vi "Lab7-PSK_Simulation_4PSK_Simple.vi"() -> ()   [LabVIEW 2013]
uses:
  <vilib>/picture/picture.llb/Draw True-Color Pixmap.vi
  <vilib>/addons/Modulation/Digital/General/MT Generate Bits (Galois, PN Order).vi
  <vilib>/addons/Modulation/Digital/General/MT Generate PSK System Parameters(M).vi
  <vilib>/addons/Modulation/Digital/General/MT Generate PSK Synchronization Parameters (bit array).vi
  <vilib>/addons/Modulation/Digital/General/MT Format Eye Diagram (complex).vi
  <vilib>/addons/Modulation/niDMT.lvlib
panel:
  in  "?":enum32{"Constellation Plot", "Eye Diagram"}(tab)
  out "Constellation Plot":T1(graph)=[{"constellation"=[-0.6843393450045908, -0.7188173867833647, -0.6862679721424542, -0.7297030487459608, -0.7159912856499204, 0.7221248350001428, -0.69319374455267, -0.7177933374862676, 0.6893145049073991, 0.7164949508669772, -0.7136233597527977, 0.7088022813066004, 0.7026806753460019, 0.6993908820448104, 0.7033303803758204, 0.7023239283689477, -0.7092821972958672, 0.7043694263023035, -0.71123073342578, -0.7063013580615412, 0.7025174893431778, -0.7079249457114573, 0.7056952690720733, -0.711060440916994, -0.7135916049305011, -0.7042966683375681, -0.7053639500078486, -0.7170793110386893, 0.7007122470722706, -0.7041907238690962, 0.7069307076270948, -0.7303032352912369, 0.7036742608538313, -0.7213763894899665, 0.6974920430188264, -0.6906276182534745, 0.7110338385529501, 0.707668395707459, 0.7066450908567875, 0.7156573983712801, 0.7058430026446071, 0.7226424194495579, -0.6941394170921843, 0.7153952742388731, -0.7061754291757949, 0.6989077999376425, 0.7322949703863137, -0.7277124364880128, 0.7152053555332901, -0.7144386806873485, 0.7122523333502172, -0.6946532350705298, -0.6977995339788963], "oversampled data"=[-0.6885507056398621, -0.6904021301332153, -0.701720009748651, 0.7230147663617461, 0.6792985003415442, 0.714980330495899, 0.7083798924531897, -0.7030264642885489, 0.7016069656212314, -0.6995735246622811, -0.7187083014951974, 0.718556461974981, -0.7154964369422703, -0.7143626925937305, -0.7168215682367294, 0.6901290658424636, 0.7193430662186729, 0.7021618219264352, -0.7044915371643418, 0.7010427354068245, 0.72862911894502, -0.6931780204687834, -0.7208414620302925, 0.6898461638663613, 0.7171050214665211, 0.7071101521691305, -0.7158811583840712, 0.7100771986297291, 0.7055043383295747, 0.7197934468495215, -0.7126751015343431, 0.699715799910657, 0.7071055136917425, 0.7000396806158872, 0.6959369636505729, 0.7171363071737368, 0.7097950846368283, 0.707670861017943, 0.6989567675175453, -0.7157042609479739, 0.7040676123623458, 0.7131191099779645, 0.7010491472655718, 0.7001052143691281, -0.7044803945850813, 0.6953086657664377, 0.7183481414573912, 0.7015721146800344, -0.6848840235343148, -0.712341720231345, 0.7005395668208682, 0.6964886799304421, 0.6911618122252481]}, {"constellation"=array[848 elements], "oversampled data"=array[848 elements]}]
  out "Eye Diagram":cluster{"t0":dbl, "dt":dbl, "Y":dbl[]}[](graph)
  out "Recovered Image":picture
  out "Transmitted Image":picture
  in  "path to JPEG file":path=path "D:/wendy/study/2023-2024Spring/EE206lab/lab7/smiley_tiny(recomended).jpg"
  out "sync found index (symbols)":dbl format="%.4f"
  in  "Eb/N0 (dB)":dbl(slide)=48.26086956521739 scale=-10.0..50.0
  out "measurements":T2 caption="Measurements" {"phase offset (deg)" format="%.2f"; "frequency drift (Hz)" format="%.2f"; "frequency offset (Hz)" format="%.2f"}
  out "Baseband Waveform":cluster{"t0":dbl, "dt":dbl, "Y":dbl[]}(graph)
  in  "M-PSK (4)":i32=4
  out "LED Array":T3
  out "error out":errorcluster
  in  "stop 2":bool
  # "M-PSK Simulation"
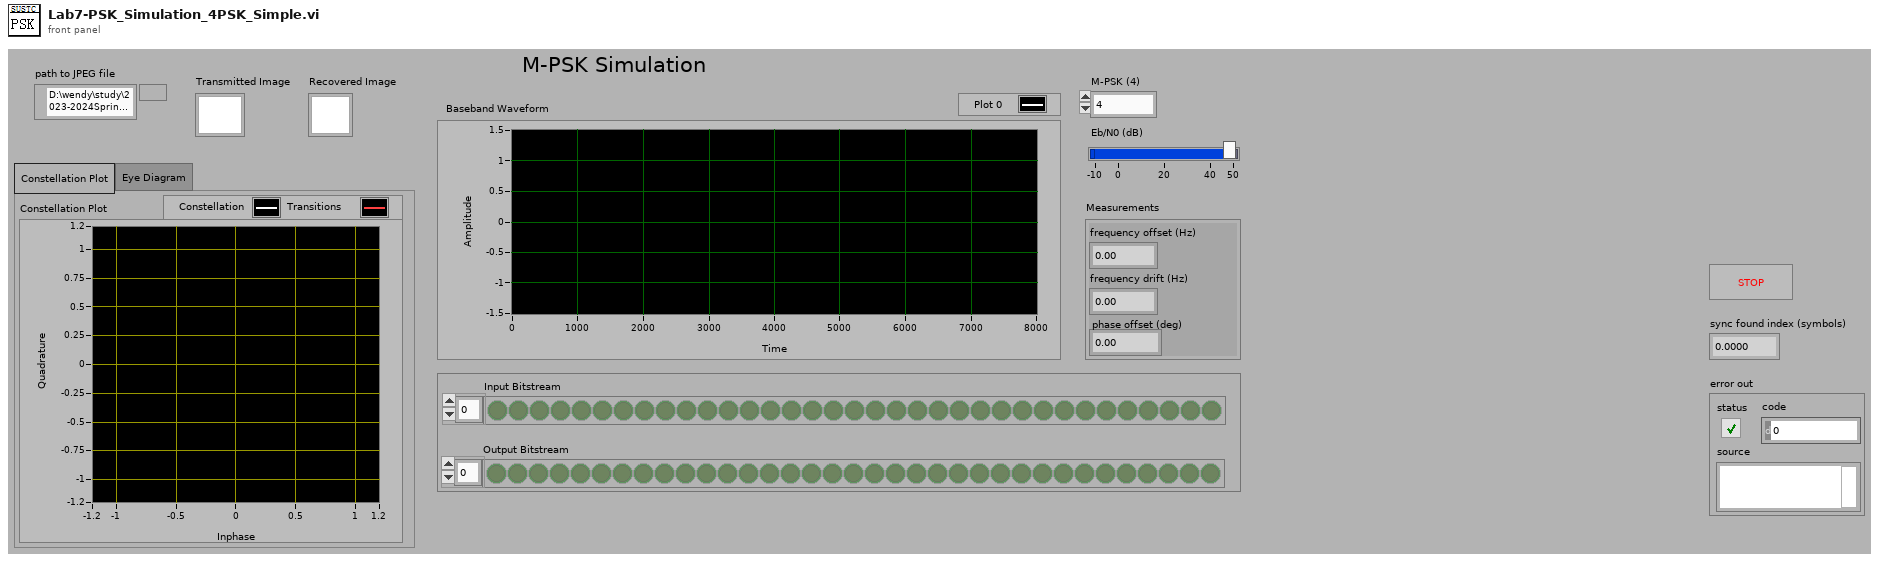
[diagram p1: front panel]
types:
  T1 = cluster{"constellation":dbl[], "oversampled data":dbl[]}[]
  T2 = cluster{"frequency offset (Hz)":dbl, "frequency drift (Hz)":dbl, "phase offset (deg)":dbl}
  T3 = cluster{"Input Bitstream":bool[], "Output Bitstream":bool[]}
  T4 = typedef "imagedata.ctl" = cluster{"image type":i32, "image depth":i32, "image":u8[], "mask":u8[], "colors":u32[], "Rectangle":cluster{"left":i16, "top":i16, "right":i16, "bottom":i16}}
  T5 = enum16{"none", "Raised Cosine", "Root Raised Cos", "Gaussian"}
  T6 = enum16{"FSK", "PSK", "QAM", "MSK", "PAM", "ASK", "CPM"}
  T7 = cluster{"samples per symbol (16)":i32, "symbol map":cdb[], "differential PSK":enum16{"disable", "enable"}, "PSK type":u16}
  T8 = typedef "niAMT.lvlib/Complex Data Waveform.ctl" = cluster{"t0":dbl, "dt":dbl, "Y":cdb[]}
  T9 = cluster{"expected sync location (symbols)":i32, "sync sequence":cdb[], "sync location uncertainty (symbols)":i32, "sync indent (symbols)":i32}
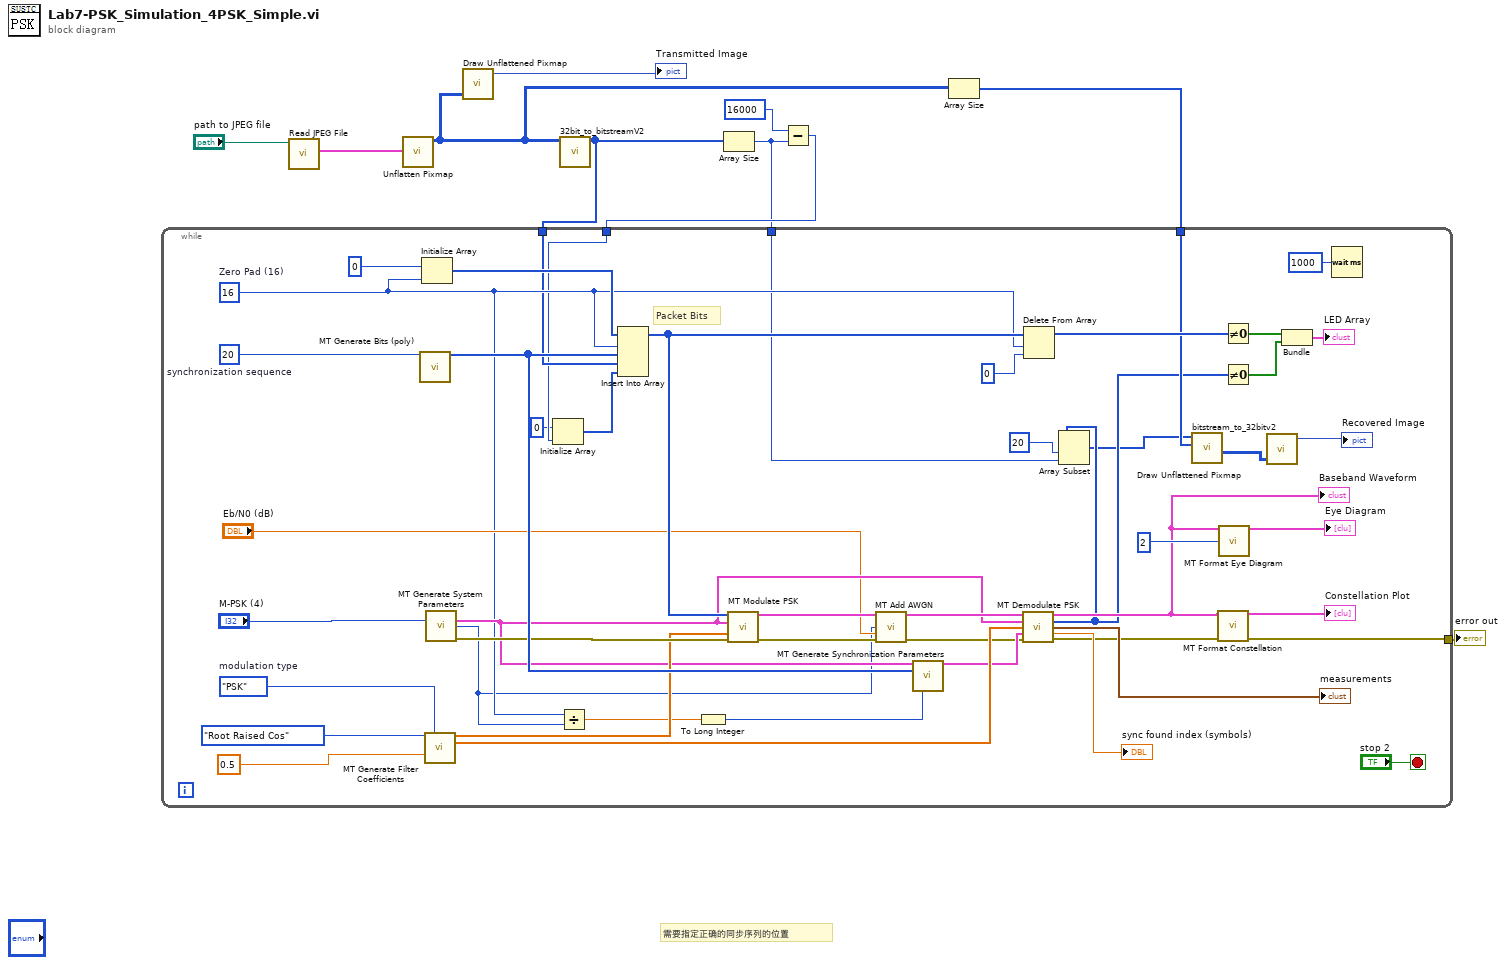
[diagram p0: block diagram]
diagram:
  # "需要指定正确的同步序列的位置"
  n1 = call <vilib>:"Read JPEG File.vi"("path to JPEG file"="path to JPEG file") -> ("image data"=w9:T4)  [unwired: 8 in, 2 out]
  n2 = call <vilib>:"Unflatten Pixmap.vi"("image data"=w9) -> ("24-bit pixmap"=w3:u32[][])  [unwired: 4 in, 6 out]
  n3 = call-poly <vilib>:"Draw Unflattened Pixmap.vi"("data (RGB format)"=w3) -> ("new picture"=→"Transmitted Image":picture)  [unwired: 8 in]
  n4 = call "32bit_to_bitstreamV2.vi"("24-bit pixmap"=w3) -> ("Bitstream with Guard"=w6:u8[])  [unwired: 7 in, 1 out]
  n5 = Array Size(array=w6) -> (size(s)=w1:i32)
  n6 = Subtract(x=16000, y=w1) -> (x-y=w4:i32)
  n7 = Array Size(array=w3) -> (size(s)=w2:i32[])
  n8 = while {
    tunnel: [w15] -> w10
    tunnel: w6 -> [w27]
    tunnel: w4 -> [w25]
    tunnel: w2 -> [w23]
    tunnel: w1 -> [w11]
    stop <- "stop 2" stop-if-true
    w31 = 16  # Zero Pad (16)
    w53 = 20  # synchronization sequence
    w59 = T6."PSK"  # modulation type
    # "Packet Bits"
    n9 = call-poly <vilib>:"MT Generate Bits (poly).vi"("total bits (128)"=w53) -> ("output bit stream"=w49:i8[])  [unwired: 12 in, 2 out]
    n10 = Initialize Array(i8 0 ("element"), w31) -> (w46:i8[])
    n11 = call <vilib>:"MT Generate Filter Coefficients.vi"("pulse shaping filter (none)"=T5."Root Raised Cos", "modulation type"=w59, "filter parameter"=0.5) -> ("pulse shaping filter coefficients"=w40:dbl[], "matched filter coefficients"=w54:dbl[])  [unwired: 10 in, 1 out]
    n12 = call-poly <vilib>:"MT Generate System Parameters.vi"("M-PSK (4)"="M-PSK (4)") -> ("PSK system parameters"=w36:T7, "bits per symbol"=w28:i32, "error out"=w44:errorcluster)  [unwired: 12 in]
    n13 = Initialize Array(0 ("element"), w25) -> (w26:i32[])
    n14 = Divide(x=w31, y=w28) -> (x/y=w30:dbl)
    n15 = Insert Into Array(array=w46, index=w31, new element #1=w49, new element #2=w27, new element #3=w26) -> (w52:i8[])
    n16 = To Long Integer(number=w30) -> (32bit integer=w29:i32)
    n17 = call <vilib>:"MT Modulate PSK.vi"("input bit stream"=w52, "PSK system parameters"=w36, "pulse shaping filter coefficients"=w40, "error in (no error)"=w44) -> ("output complex waveform"=w39:T8, "error out"=w34:errorcluster)  [unwired: 9 in, 1 out]
    n18 = call <vilib>:"MT Add AWGN.vi"("input complex waveform"=w39, "bits per symbol (1)"=w28, "Eb/N0 (10 dB)"="Eb/N0 (dB)", "error in (no error)"=w34) -> ("output complex waveform"=w38:T8, "error out"=w35:errorcluster)  [unwired: 9 in, 1 out]
    n19 = call-poly <vilib>:"MT Generate Synchronization Parameters.vi"("PSK system parameters"=w36, "sync bits"=w49, "expected sync location (symbols)"=w29) -> ("PSK synchronization parameters"=w48:T9)  [unwired: 11 in, 1 out]
    n20 = call <vilib>:"MT Demodulate PSK.vi"("input complex waveform"=w38, "PSK system parameters"=w36, "matched filter coefficients"=w54, "synchronization parameters"=w48, "error in (no error)"=w35) -> ("recovered complex waveform"=w17:T8, "output bit stream"=w13:i8[], "measurements"=→"measurements":T2, "sync found index (symbols)"=→"sync found index (symbols)":dbl, "error out"=w16:errorcluster)  [unwired: 6 in]
    "Baseband Waveform" <- w17
    n21 = Delete From Array(array=w52, length=w31, index=0) -> (array with subset deleted=w50:i8[])  [unwired: 1 out]
    n22 = Array Subset(array=w13, index=20 ("length"), length=w11) -> (w12:i8[])
    n23 = call "bitstream_to_32bitv2.vi"("JPG Size"=w23, "Bitstream Input"=w12) -> ("2D JPG Array"=w22:u32[][])  [unwired: 8 in, 1 out]
    n24 = call <vilib>:"MT Format Constellation.vi"("waveform"=w17, "error in (no error)"=w16) -> ("constellation graph"=→"Constellation Plot":T1, "error out"=w15:errorcluster)  [unwired: 12 in]
    n25 = call-poly <vilib>:"MT Format Eye Diagram.vi"("waveform"=w17, "eye length"=2) -> ("eye diagram"=→"Eye Diagram":cluster{"t0":dbl, "dt":dbl, "Y":dbl[]}[])  [unwired: 12 in, 1 out]
    n26 = Not Equal To 0?(x=w50) -> (x != 0?=w57:bool[])
    n27 = Not Equal To 0?(x=w13) -> (x != 0?=w56:bool[])
    n28 = call-poly <vilib>:"Draw Unflattened Pixmap.vi"("data (RGB format)"=w22) -> ("new picture"=→"Recovered Image":picture)  [unwired: 8 in]
    n29 = Bundle(w57, w56) -> (→"LED Array":cluster{bool[], bool[]})  [unwired: 1 in]
    n30 = Wait (ms)(milliseconds to wait=u32 1000) -> ()  [unwired: 1 out]
  }
  "error out" <- w10
